vi "Post action.vi"(6 "Index":i32=41, 8 "error in (no error)":errorcluster, 9 "PostAction":T1, 11 "SweepControl":refnum<class "SweepControl.lvclass">) -> (0 "error out":errorcluster, 3 "SweepControl":refnum<class "SweepControl.lvclass">)   [LabVIEW 2019, in "SweepControl.lvclass"]
uses:
  SweepControl.lvclass
  <userlib>/LevyLab/Levylab Instruments/Instrument Types/Cryostat/Instrument.Cryostat.lvclass
  Control Experiment/Control Experiment.lvclass
  Transport/Transport.lvclass
  Typedefs/Enum - PostAction.ctl
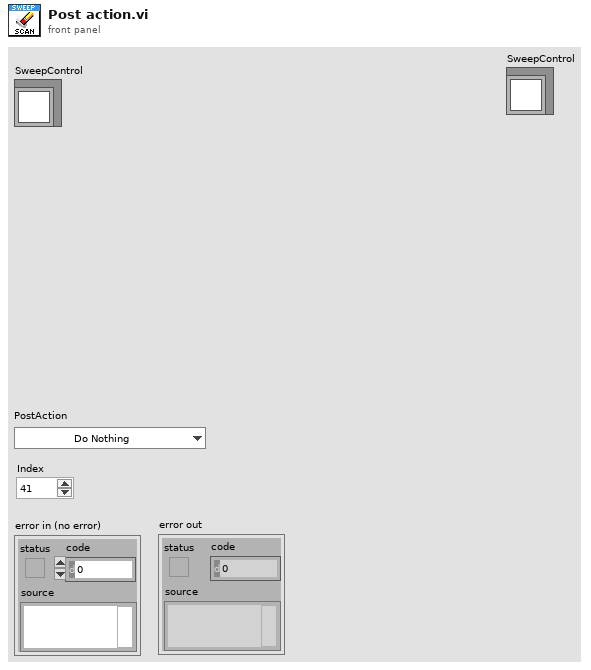
[diagram p1: front panel]
types:
  T1 = typedef "SweepControl.lvclass/Enum - PostAction.ctl" = enum16{"Do Nothing", "Wait (time)", "Wait (Temperature)", "Wait (<T ; B sweep)", "Wait (Magnet)"}
  T2 = typedef "SweepControl.lvclass/Cluster - ScanParamters.ctl" = cluster{"Start":dbl, "End":dbl, "Step":dbl, "Rate":dbl, "Waveform type":enum16{"linear", "triangle", "power"}, "wait (ms or K)":dbl, "Address":string, "channel":i32}
  T3 = typedef "Control Experiment.lvclass/Instruments--cluster.ctl" = cluster{"KH7008":refnum<class "Instrument.KH7008.lvclass">[], "Lockin":refnum<class "Instrument.Lockin.lvclass">, "Temperature":refnum<class "Instrument.Cryostat.lvclass">, "Magnet":refnum<class "Instrument.Cryostat.lvclass">, "Rotator":refnum<class "Instrument.Cryostat.lvclass">, "Level":refnum<class "Instrument.Cryostat.lvclass">, "Capacitance Bridge":refnum<class "Instrument.CBridge.lvclass">, "Delay Line":refnum<class "Instrument.DelayLine.lvclass">, "Strain Cell":refnum<class "Instrument.Strain.lvclass">, "VNA":refnum<class "Instrument.VNA.lvclass">, "Voltage Source":refnum<class "Instrument.VSource.lvclass">}
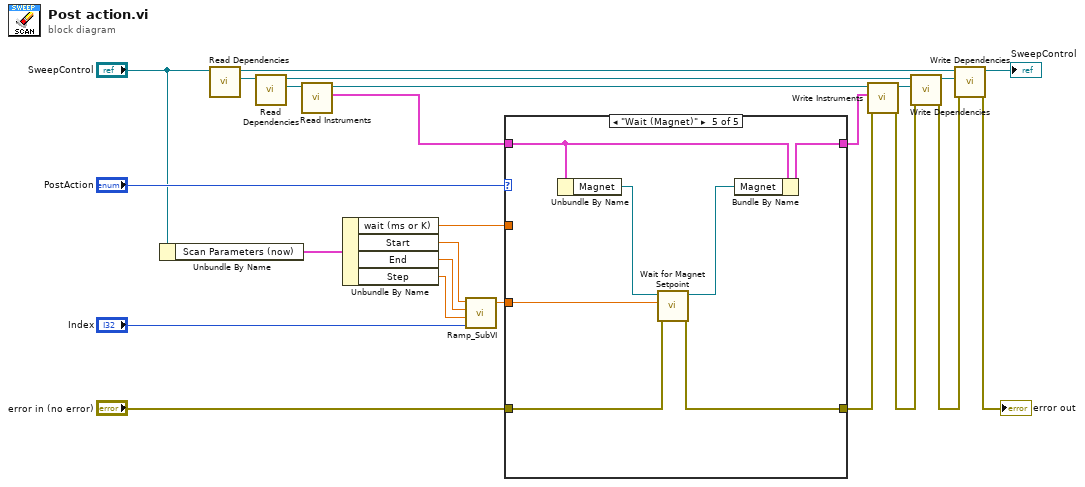
[diagram p0: block diagram]
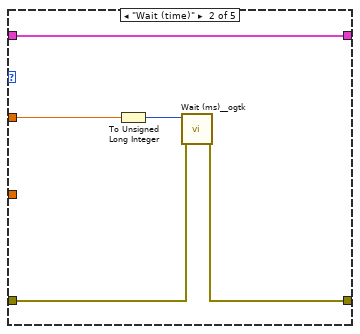
[diagram p3: hidden frame]
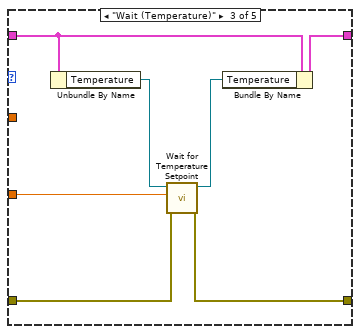
[diagram p4: hidden frame]
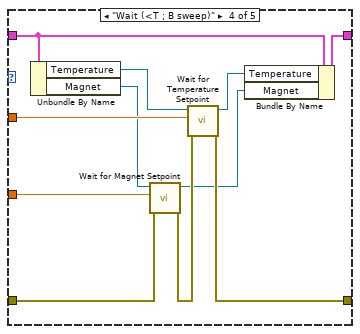
[diagram p5: hidden frame]
diagram:
  n1 = Unbundle By Name("SweepControl") -> ("Scan Parameters (now)"=w16:T2)
  n2 = call "Read Dependencies.vi"("SweepControl in"="SweepControl") -> ("Transport"=w10:refnum<class "Transport.lvclass">, "SweepControl out"=w3:refnum<class "SweepControl.lvclass">)  [unwired: 8 in, 1 out]
  n3 = call "Read Dependencies.vi"("Transport"=w10) -> ("C.E."=w11:refnum<class "Control Experiment.lvclass">, "Transport"=w5:refnum<class "Transport.lvclass">)  [unwired: 8 in, 1 out]
  n4 = call "Read Instruments.vi"("Control Experiment in"=w11) -> ("Instruments"=w17:T3, "Control Experiment out"=w4:refnum<class "Control Experiment.lvclass">)  [unwired: 8 in, 1 out]
  n5 = Unbundle By Name(w16) -> ("wait (ms or K)"=w18:dbl, "Start"=w21:dbl, "End"=w20:dbl, "Step"=w19:dbl)
  n6 = call <userlib>:"Ramp_SubVI.vi"("index"="Index", "step"=w19, "end"=w20, "start"=w21) -> ("Numeric"=w23:dbl)  [unwired: 1 in, 1 out]
  n7 = case shown="\"Wait (Magnet)\"" "PostAction" {
    tunnel: w23 -> [_ _ w38 w47 w56]
    tunnel: w18 -> [_ w31 _ w48 _]
    tunnel: "error in (no error)" -> [w26 w30 w37 w46 w55]
    tunnel: [w26 w29 w36 w49 w54] -> w13
    tunnel: w17 -> [w25 w27 w34 w43 w52]
    tunnel: [w25 w27 w32 w41 w50] -> w14
    frame "Do Nothing", Default {
    }
    frame "Wait (time)" {
      n8 = To Unsigned Long Integer(number=w31) -> (unsigned 32bit integer=w28:u32)
      n9 = call <userlib>:"Wait (ms)__ogtk.vi"("error in (no error)"=w30, "milliseconds to wait"=w28) -> ("error out"=w29:errorcluster)  [unwired: 8 in, 1 out]
    }
    frame "Wait (Temperature)" {
      n10 = Unbundle By Name(w34) -> ("Temperature"=w35:refnum<class "Instrument.Cryostat.lvclass">)
      n11 = call <userlib>:"Wait for Temperature Setpoint.vi"("error in (no error)"=w37, "Setpoint (K)"=w38, "Instrument.Cryostat in"=w35) -> ("error out"=w36:errorcluster, "Instrument.Cryostat out"=w33:refnum<class "Instrument.Cryostat.lvclass">)  [unwired: 7 in]
      n12 = Bundle By Name(cluster=w34, "Temperature"=w33) -> (w32:T3)
    }
    frame "Wait (<T ; B sweep)" {
      n13 = Unbundle By Name(w43) -> ("Temperature"=w39:refnum<class "Instrument.Cryostat.lvclass">, "Magnet"=w44:refnum<class "Instrument.Cryostat.lvclass">)
      n14 = call <userlib>:"Wait for Magnet Setpoint.vi"("error in (no error)"=w46, "Setpoint (T)"=w47, "Instrument.Cryostat in"=w44) -> ("error out"=w45:errorcluster, "Instrument.Cryostat out"=w42:refnum<class "Instrument.Cryostat.lvclass">)  [unwired: 7 in]
      n15 = call <userlib>:"Wait for Temperature Setpoint.vi"("error in (no error)"=w45, "Setpoint (K)"=w48, "Instrument.Cryostat in"=w39) -> ("error out"=w49:errorcluster, "Instrument.Cryostat out"=w40:refnum<class "Instrument.Cryostat.lvclass">)  [unwired: 7 in]
      n16 = Bundle By Name(cluster=w43, "Temperature"=w40, "Magnet"=w42) -> (w41:T3)
    }
    frame "Wait (Magnet)" {
      n17 = Unbundle By Name(w52) -> ("Magnet"=w53:refnum<class "Instrument.Cryostat.lvclass">)
      n18 = call <userlib>:"Wait for Magnet Setpoint.vi"("error in (no error)"=w55, "Setpoint (T)"=w56, "Instrument.Cryostat in"=w53) -> ("error out"=w54:errorcluster, "Instrument.Cryostat out"=w51:refnum<class "Instrument.Cryostat.lvclass">)  [unwired: 7 in]
      n19 = Bundle By Name(cluster=w52, "Magnet"=w51) -> (w50:T3)
    }
  }
  n20 = call "Write Instruments.vi"("error in (no error)"=w13, "Instruments"=w14, "Control Experiment in"=w4) -> ("error out"=w12:errorcluster, "Control Experiment out"=w15:refnum<class "Control Experiment.lvclass">)  [unwired: 7 in]
  n21 = call "Write Dependencies.vi"("error in (no error)"=w12, "Control Experiment"=w15, "Transport in"=w5) -> ("error out"=w7:errorcluster, "Transport out"=w9:refnum<class "Transport.lvclass">)  [unwired: 7 in]
  n22 = call "Write Dependencies.vi"("error in (no error)"=w7, "Transport"=w9, "SweepControl in"=w3) -> ("error out"=→"error out":errorcluster, "SweepControl out"=→"SweepControl":refnum<class "SweepControl.lvclass">)  [unwired: 7 in]
